vi "Demultiplexer.vi"() -> ()   [LabVIEW 2021]
panel:
  out "Y3":bool
  out "Y2":bool
  out "Y1":bool
  out "Y0":bool
  in  "S1":bool
  in  "S0":bool
  in  "Input":bool
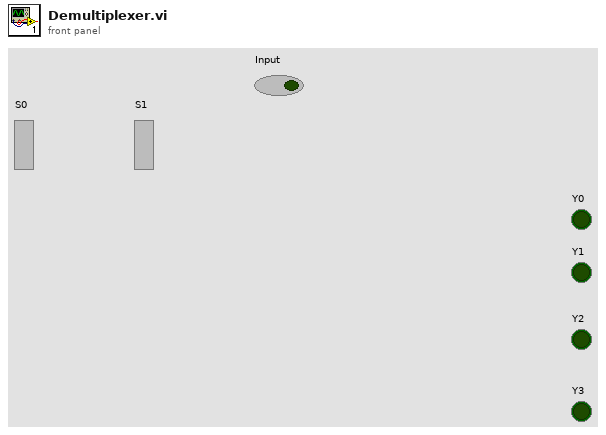
[diagram p1: front panel]
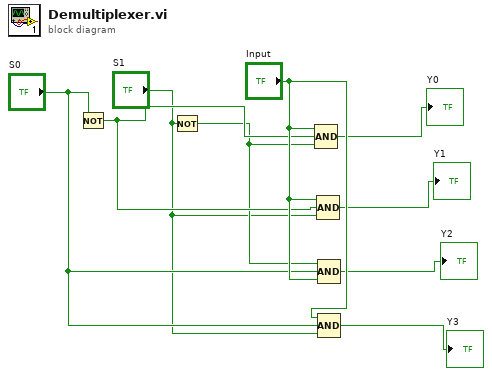
[diagram p0: block diagram]
diagram:
  n1 = Not(x="S0") -> (.not. x?=w4:bool)
  n2 = Not(x="S1") -> (.not. x?=w3:bool)
  n3 = Compound Arithmetic op=AND("Input", w4, w3) -> (→"Y0":bool)
  n4 = Compound Arithmetic op=AND("Input", w4, "S1") -> (→"Y1":bool)
  n5 = Compound Arithmetic op=AND(w3, "S0", "Input") -> (→"Y2":bool)
  n6 = Compound Arithmetic op=AND("Input", "S0", "S1") -> (→"Y3":bool)
